vi "test_GetItemInfosFromProjectFile_TargetsDifferentCompilersAdvancedPPLSolution.vi"() -> (3 "Pass?":bool)   [LabVIEW 2019, in "Tests.SolutionBuilder.lvlib"]
uses:
  Tests.SolutionBuilder.lvlib
  SolutionBuilder/SolutionBuilder.lvclass
  SolutionBuilder/ProjectItem/ProjectItem.lvclass
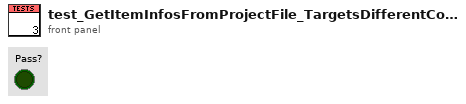
[diagram p1: front panel]
types:
  T1 = typedef "SolutionBuilder.lvlib/SolutionBuilder.lvclass/ProjectItemMap.ctl" = map{path, refnum<class "ProjectItem.lvclass">[]}
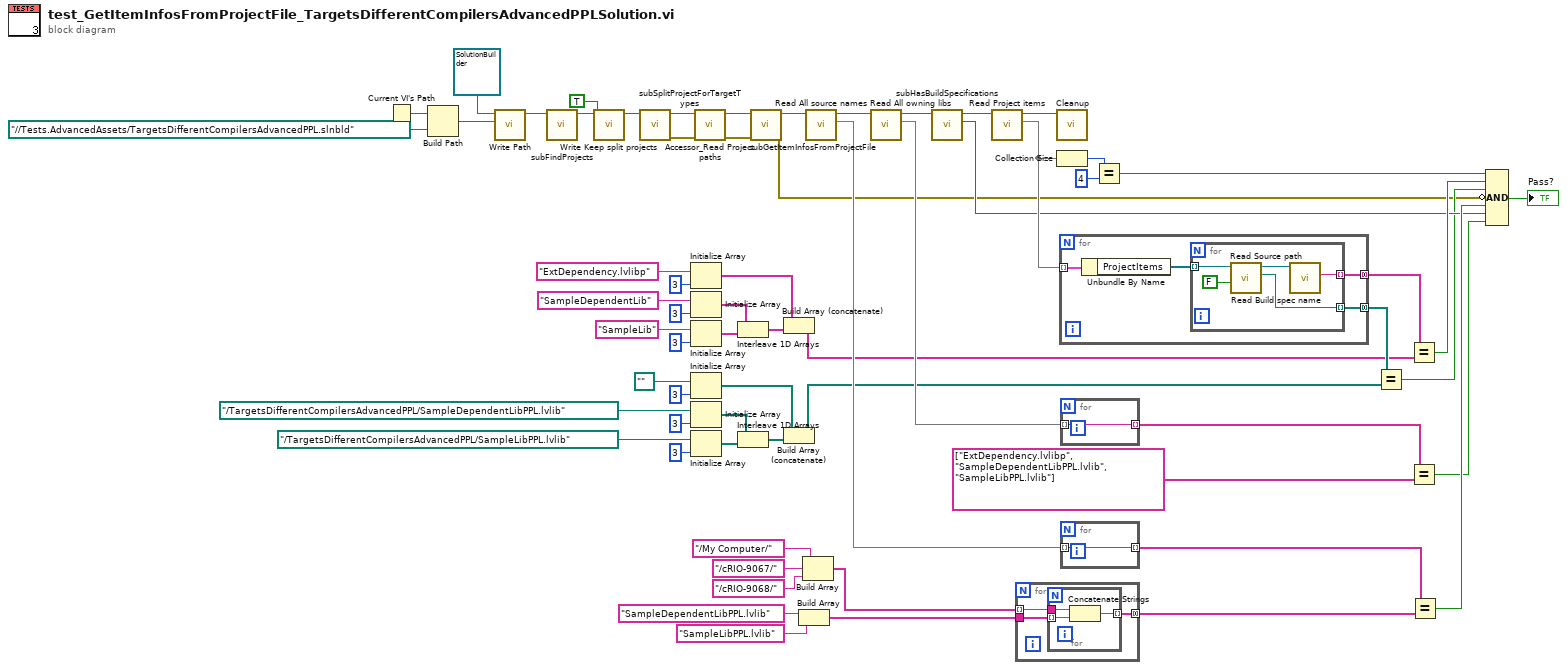
[diagram p0: block diagram]
diagram:
  n1 = Current VI's Path() -> (path=w63:path)
  n2 = Build Path(base path=w63, name or relative path=path "../../Tests.AdvancedAssets/TargetsDifferentCompilersAdvancedPPL.slnbld" ("Path")) -> (appended path=w61:path)
  n3 = call "Write Path.vi"("Path"=w61, "SolutionBuilder in"=refnum<class "SolutionBuilder.lvclass"> refnum) -> ("SolutionBuilder out"=w64:refnum<class "SolutionBuilder.lvclass">)  [unwired: 9 in]
  n4 = call "subFindProjects.vi"("SolutionBuilder in"=w64) -> ("SolutionBuilder out"=w3:refnum<class "SolutionBuilder.lvclass">)  [unwired: 9 in, 1 out]
  n5 = call-dynamic "Write Keep split projects.vi"("Keep split projects?"=TRUE, "SolutionBuilder in"=w3) -> ("SolutionBuilder out"=w2:refnum<class "SolutionBuilder.lvclass">)  [unwired: 9 in]
  n6 = call "subSplitProjectForTargetTypes.vi"("SolutionBuilder in"=w2) -> ("error out"=w6:errorcluster, "SolutionBuilder out"=w7:refnum<class "SolutionBuilder.lvclass">)  [unwired: 9 in]
  n7 = Initialize Array("ExtDependency.lvlibp" ("Build spec name"), 3 ("dimension size")) -> (w30:string[])
  n8 = Initialize Array("SampleDependentLib" ("Build spec name"), 3 ("dimension size")) -> (w33:string[])
  n9 = Initialize Array("SampleLib" ("Build spec name"), 3 ("dimension size")) -> (w32:string[])
  n10 = Initialize Array(path "" ("Source path"), 3 ("dimension size")) -> (w28:path[])
  n11 = Initialize Array(path "../TargetsDifferentCompilersAdvancedPPL/SampleDependentLibPPL.lvlib" ("Source path"), 3 ("dimension size")) -> (w25:path[])
  n12 = Initialize Array(path "../TargetsDifferentCompilersAdvancedPPL/SampleLibPPL.lvlib" ("Source path"), 3 ("dimension size")) -> (w26:path[])
  n13 = call "Accessor_Read Project paths.vi"("error in (no error)"=w6, "SolutionBuilder in"=w7) -> ("error out"=w4:errorcluster, "SolutionBuilder out"=w5:refnum<class "SolutionBuilder.lvclass">)  [unwired: 7 in, 1 out]
  n14 = Interleave 1D Arrays(w33, w32) -> (w31:string[])
  n15 = Interleave 1D Arrays(w25, w26) -> (w27:path[])
  n16 = call "subGetItemInfosFromProjectFile.vi"("error in (no error)"=w4, "SolutionBuilder in"=w5) -> ("error out"=w40:errorcluster, "SolutionBuilder out"=w58:refnum<class "SolutionBuilder.lvclass">)  [unwired: 8 in]
  n17 = Build Array (concatenate)(w30, w31) -> (w29:string[])
  n18 = Build Array (concatenate)(w28, w27) -> (w18:path[])
  n19 = Build Array("SampleDependentLibPPL.lvlib" ("Build spec name"), "SampleLibPPL.lvlib" ("Build spec name")) -> (w11:string[])
  n20 = Build Array("/My Computer/" ("Build spec name"), "/cRIO-9067/" ("Build spec name"), "/cRIO-9068/" ("Build spec name")) -> (w12:string[])
  n21 = call "Read All source names.vi"("SolutionBuilder in"=w58) -> ("All source names"=w54:set{string}, "SolutionBuilder out"=w46:refnum<class "SolutionBuilder.lvclass">)  [unwired: 9 in]
  n22 = call "Read All owning libs.vi"("SolutionBuilder in"=w46) -> ("All owning libs"=w44:set{string}, "SolutionBuilder out"=w45:refnum<class "SolutionBuilder.lvclass">)  [unwired: 9 in]
  n23 = call "subHasBuildSpecifications.vi"("SolutionBuilder in"=w45) -> ("Has specs?"=w51:bool, "SolutionBuilder out"=w52:refnum<class "SolutionBuilder.lvclass">)  [unwired: 8 in, 1 out]
  n24 = call "Read Project items.vi"("SolutionBuilder in"=w52) -> ("Project items"=w57:T1, "SolutionBuilder out"=w8:refnum<class "SolutionBuilder.lvclass">)  [unwired: 9 in]
  n25 = for {
    tunnel: w12 -> [w68] mode=indexing
    tunnel: w11 -> [w67]
    tunnel: [w66] -> w10 mode=concatenating
    n26 = for {
      tunnel: w68 -> [w71]
      tunnel: w67 -> [w70] mode=indexing
      tunnel: [w69] -> w66 mode=indexing
      n27 = Concatenate Strings(w71, w70) -> (w69:string)
    }
  }
  n28 = call "Cleanup.vi"("SolutionBuilder in"=w8) -> ()  [unwired: 9 in, 2 out]
  n29 = Collection Size(1:w57) -> (0:w60:i32)
  n30 = for {
    tunnel: w57 -> [w75] mode=indexing
    tunnel: [w74] -> w50 mode=concatenating
    tunnel: [w72] -> w48 mode=concatenating
    n31 = Unbundle By Name(w75) -> ("ProjectItems"=w73:refnum<class "ProjectItem.lvclass">[])
    n32 = for {
      tunnel: w73 -> [w78] mode=indexing
      tunnel: [w80] -> w74 mode=indexing
      tunnel: [w77] -> w72 mode=indexing
      n33 = call "Read Source path.vi"("Force abs path? (T)"=FALSE, "ProjectItem in"=w78) -> ("Source path"=w77:path, "ProjectItem out"=w79:refnum<class "ProjectItem.lvclass">)  [unwired: 8 in]
      n34 = call "Read Build spec name.vi"("ProjectItem in"=w79) -> ("Build spec name"=w80:string)  [unwired: 9 in, 1 out]
    }
  }
  n35 = for {
    tunnel: w44 -> [w81] mode=indexing
    tunnel: [w81] -> w43 mode=indexing
  }
  n36 = for {
    tunnel: w54 -> [w82] mode=indexing
    tunnel: [w82] -> w49 mode=indexing
  }
  n37 = Equal?(x=w60, y=4) -> (x = y?=w56:bool)
  n38 = Equal?(x=w48, y=w18) -> (x = y?=w47:bool)
  n39 = Equal?(x=w50, y=w29) -> (x = y?=w55:bool)
  n40 = Equal?(x=w43, y=string[] ["ExtDependency.lvlibp", "SampleDependentLibPPL.lvlib", "SampleLibPPL.lvlib"] ("Array")) -> (x = y?=w41:bool)
  n41 = Equal?(x=w49, y=w10) -> (x = y?=w53:bool)
  n42 = Compound Arithmetic op=AND(w56, w55, w47, invert w40, w53, w51, w41) -> (→"Pass?":bool)
